vi "ParserProperties.vi"(6 "error in (no error)":errorcluster, 8 "enums":T1[](array[typedef]), 9 "JSON item":string) -> (0 "error out":errorcluster, 2 "properties":T3[](array[typedef]), 3 "JSON item":string)   [LabVIEW 2017, in "Paser.lvlib"]
uses:
  Paser.lvlib
  Ctrl/Property.ctl
  <vilib>/JDP Science/JSONtext/JSONtext.lvlib
  1cc933f8-08c6-49f7-934d-c4f15ecdcb85.vi
  e9c6c34c-2ba3-4e56-8d9d-7534e8e085fc.vi
  5c37e213-318c-4559-b132-54769381f561.vi
  7b41418e-2d6c-4ed8-9453-ba65fd8ca716.vi
  5016f5cf-20b5-4117-aa62-07d20ba2ba5b.vi
  Ctrl/EnumValue.ctl
  Ctrl/Enum.ctl
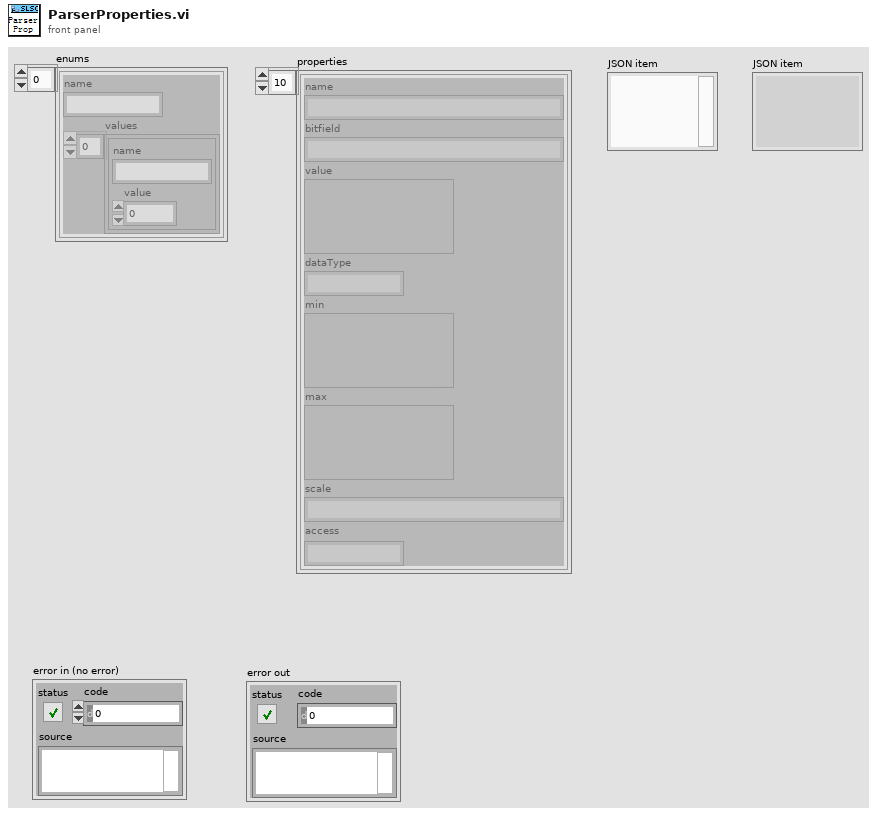
[diagram p1: front panel]
types:
  T1 = typedef "Enum.ctl" = cluster{"name":string, "values":T2[]}
  T2 = typedef "EnumValue.ctl" = cluster{"name":string, "value":i32}
  T3 = typedef "Property.ctl" = cluster{"name":string, "bitfield":string, "value":variant, "dataType":string, "min":variant, "max":variant, "scale":string, "access":string}
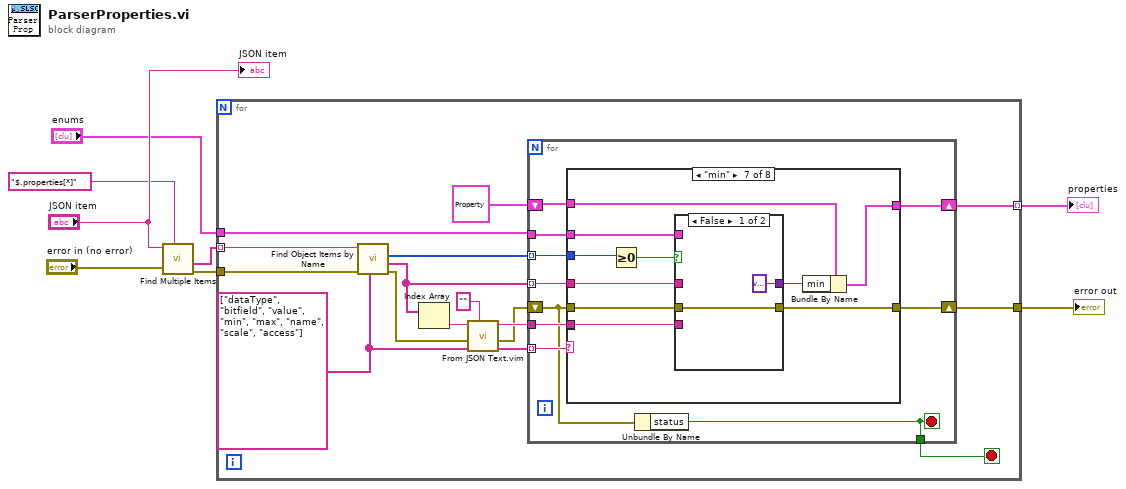
[diagram p0: block diagram]
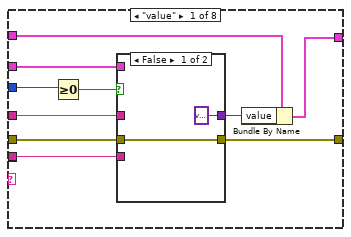
[diagram p2: hidden frame]
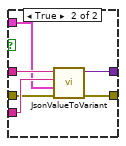
[diagram p3: hidden frame]
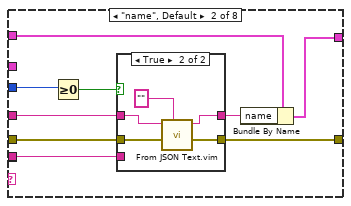
[diagram p4: hidden frame]
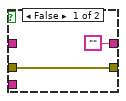
[diagram p5: hidden frame]
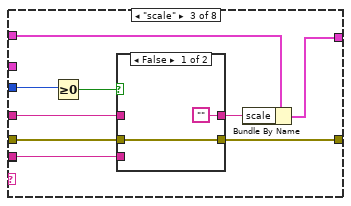
[diagram p6: hidden frame]
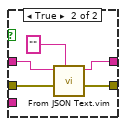
[diagram p7: hidden frame]
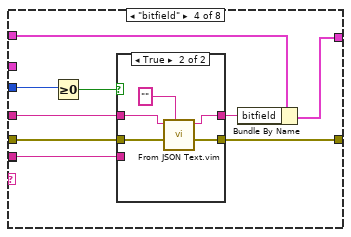
[diagram p8: hidden frame]
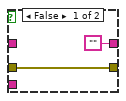
[diagram p9: hidden frame]
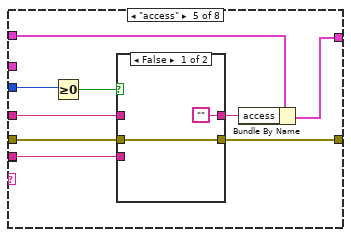
[diagram p10: hidden frame]
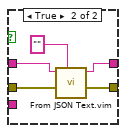
[diagram p11: hidden frame]
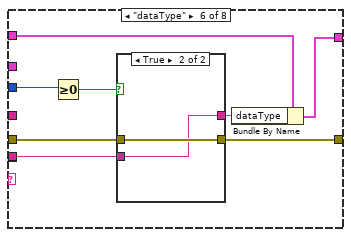
[diagram p12: hidden frame]
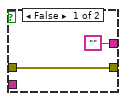
[diagram p13: hidden frame]
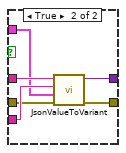
[diagram p14: hidden frame]
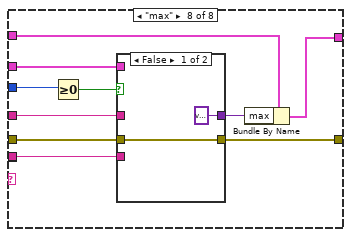
[diagram p15: hidden frame]
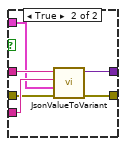
[diagram p16: hidden frame]
diagram:
  n1 = call <vilib>:"Find Multiple Items.vi"("$Path or Item Name"="$.properties[*]" ("$properties path"), "error in (no error)"="error in (no error)", "JSON"="JSON item") -> ("error out"=w3:errorcluster, "<JSON>"=w4:string[])  [unwired: 5 in, 2 out]
  n2 = for {
    tunnel: w3 -> [w22]
    tunnel: w4 -> [w23] mode=indexing
    tunnel: [w19] -> w8 mode=indexing
    tunnel: [w11] -> w2
    tunnel: "enums" -> [w10]
    stop <- w9 stop-if-true
    w20 = string[] ["dataType", "bitfield", "value", "min", "max", "name", "scale", "access"] ("Item Names")
    n3 = call <vilib>:"Find Object Items by Name.vi"("Item Names"=w20, "error in (no error)"=w22, "JSON"=w23) -> ("error out"=w14:errorcluster, "<JSON>"=w15:string[], "Offsets"=w21:i32[])  [unwired: 6 in]
    n4 = Index Array(array=w15) -> (element=w18:string)  [unwired: 1 in]
    n5 = call "From JSON Text.vim"("Data Type and Default Value"="" ("element"), "error in (no error)"=w14, "JSON"=w18) -> ("error out"=w13:errorcluster, "Data out"=w16:string)  [unwired: 7 in]
    n6 = for {
      tunnel: w21 -> [w30] mode=indexing
      tunnel: w20 -> [w33] mode=indexing
      shift-right: [w31] -> w19
      shift-left: T3 {"name"="", "bitfield"="", "value"=variant, "dataType"="", "min"=variant, "max"=variant, "scale"="", "access"=""} -> [w32]
      tunnel: w15 -> [w29] mode=indexing
      tunnel: w16 -> [w28]
      shift-right: [w27] -> w11
      shift-left: w13 -> [w25]
      tunnel: w10 -> [w26]
      tunnel: [w24] -> w9
      stop <- w24 stop-if-true
      n7 = case shown="\"min\"" w33 {
        tunnel: w32 -> [w41 w58 w74 w90 w106 w122 w135 w153]
        tunnel: [w39 w57 w73 w89 w105 w121 w133 w151] -> w31
        tunnel: w30 -> [w38 w56 w72 w88 w104 w120 w132 w150]
        tunnel: w29 -> [w43 w60 w76 w92 w108 _ w137 w155]
        tunnel: [w42 w59 w75 w91 w107 w123 w136 w154] -> _
        tunnel: w28 -> [w42 w59 w75 w91 w107 w123 w136 w154]
        tunnel: w25 -> [w36 w53 w69 w85 w101 w117 w130 w148]
        tunnel: [w35 w52 w68 w84 w100 w116 w129 w147] -> w27
        tunnel: w26 -> [w34 _ _ _ _ _ w128 w146]
        frame "value" {
          n8 = Greater Or Equal To 0?(x=w38) -> (x >= 0?=w37:bool)
          n9 = case shown="False" w37 {
            tunnel: w43 -> [_ w51]
            tunnel: w42 -> [_ w50]
            tunnel: [variant ("Variant") w49] -> w40
            tunnel: w36 -> [w44 w48]
            tunnel: [w44 w47] -> w35
            tunnel: w34 -> [_ w46]
            frame False {
            }
            frame True {
              n10 = call "JsonValueToVariant.vi"("error in (no error)"=w48, "enums"=w46, "data type"=w50, "JSON item"=w51) -> ("error out"=w47:errorcluster, "Variant"=w49:variant)  [unwired: 6 in]
            }
          }
          n11 = Bundle By Name(cluster=w41, "value"=w40) -> (w39:T3)
        }
        frame "name", Default {
          n12 = Greater Or Equal To 0?(x=w56) -> (x >= 0?=w55:bool)
          n13 = case shown="True" w55 {
            tunnel: w60 -> [_ w65]
            tunnel: w59 -> [_ _]
            tunnel: ["" ("<JSON>") w64] -> w54
            tunnel: w53 -> [w61 w67]
            tunnel: [w61 w66] -> w52
            frame False {
            }
            frame True {
              n14 = call "From JSON Text.vim"("Data Type and Default Value"="" ("element"), "error in (no error)"=w67, "JSON"=w65) -> ("error out"=w66:errorcluster, "Data out"=w64:string)  [unwired: 7 in]
            }
          }
          n15 = Bundle By Name(cluster=w58, "name"=w54) -> (w57:T3)
        }
        frame "scale" {
          n16 = Greater Or Equal To 0?(x=w72) -> (x >= 0?=w71:bool)
          n17 = case shown="False" w71 {
            tunnel: w76 -> [_ w81]
            tunnel: w75 -> [_ _]
            tunnel: ["" ("<JSON>") w80] -> w70
            tunnel: w69 -> [w77 w83]
            tunnel: [w77 w82] -> w68
            frame False {
            }
            frame True {
              n18 = call "From JSON Text.vim"("Data Type and Default Value"="" ("element"), "error in (no error)"=w83, "JSON"=w81) -> ("error out"=w82:errorcluster, "Data out"=w80:string)  [unwired: 7 in]
            }
          }
          n19 = Bundle By Name(cluster=w74, "scale"=w70) -> (w73:T3)
        }
        frame "bitfield" {
          n20 = Greater Or Equal To 0?(x=w88) -> (x >= 0?=w87:bool)
          n21 = case shown="True" w87 {
            tunnel: w92 -> [_ w96]
            tunnel: w91 -> [_ _]
            tunnel: ["" ("<JSON>") w95] -> w86
            tunnel: w85 -> [w93 w99]
            tunnel: [w93 w98] -> w84
            frame False {
            }
            frame True {
              n22 = call "From JSON Text.vim"("Data Type and Default Value"="" ("element"), "error in (no error)"=w99, "JSON"=w96) -> ("error out"=w98:errorcluster, "Data out"=w95:string)  [unwired: 7 in]
            }
          }
          n23 = Bundle By Name(cluster=w90, "bitfield"=w86) -> (w89:T3)
        }
        frame "access" {
          n24 = Greater Or Equal To 0?(x=w104) -> (x >= 0?=w103:bool)
          n25 = case shown="False" w103 {
            tunnel: w108 -> [_ w112]
            tunnel: w107 -> [_ _]
            tunnel: ["" ("<JSON>") w111] -> w102
            tunnel: w101 -> [w109 w115]
            tunnel: [w109 w114] -> w100
            frame False {
            }
            frame True {
              n26 = call "From JSON Text.vim"("Data Type and Default Value"="" ("element"), "error in (no error)"=w115, "JSON"=w112) -> ("error out"=w114:errorcluster, "Data out"=w111:string)  [unwired: 7 in]
            }
          }
          n27 = Bundle By Name(cluster=w106, "access"=w102) -> (w105:T3)
        }
        frame "dataType" {
          n28 = Greater Or Equal To 0?(x=w120) -> (x >= 0?=w119:bool)
          n29 = case shown="True" w119 {
            tunnel: w123 -> [_ w126]
            tunnel: ["" ("<JSON>") w126] -> w118
            tunnel: w117 -> [w124 w127]
            tunnel: [w124 w127] -> w116
            frame False {
            }
            frame True {
            }
          }
          n30 = Bundle By Name(cluster=w122, "dataType"=w118) -> (w121:T3)
        }
        frame "min" {
          n31 = Greater Or Equal To 0?(x=w132) -> (x >= 0?=w131:bool)
          n32 = case shown="False" w131 {
            tunnel: w137 -> [_ w145]
            tunnel: w136 -> [_ w144]
            tunnel: [variant ("Variant") w143] -> w134
            tunnel: w130 -> [w138 w142]
            tunnel: [w138 w141] -> w129
            tunnel: w128 -> [_ w140]
            frame False {
            }
            frame True {
              n33 = call "JsonValueToVariant.vi"("error in (no error)"=w142, "enums"=w140, "data type"=w144, "JSON item"=w145) -> ("error out"=w141:errorcluster, "Variant"=w143:variant)  [unwired: 6 in]
            }
          }
          n34 = Bundle By Name(cluster=w135, "min"=w134) -> (w133:T3)
        }
        frame "max" {
          n35 = Greater Or Equal To 0?(x=w150) -> (x >= 0?=w149:bool)
          n36 = case shown="False" w149 {
            tunnel: w155 -> [_ w163]
            tunnel: w154 -> [_ w162]
            tunnel: [variant ("Variant") w161] -> w152
            tunnel: w148 -> [w156 w160]
            tunnel: [w156 w159] -> w147
            tunnel: w146 -> [_ w158]
            frame False {
            }
            frame True {
              n37 = call "JsonValueToVariant.vi"("error in (no error)"=w160, "enums"=w158, "data type"=w162, "JSON item"=w163) -> ("error out"=w159:errorcluster, "Variant"=w161:variant)  [unwired: 6 in]
            }
          }
          n38 = Bundle By Name(cluster=w153, "max"=w152) -> (w151:T3)
        }
      }
      n39 = Unbundle By Name(w25) -> ("status"=w24:bool)
    }
  }
  "properties" <- w8
  "error out" <- w2
  "JSON item" <- "JSON item"
